vi "query_components.vi"(8 "error in (no error)":errorcluster, 9 "version":i32, 10 "part":string, 11 "DB Session ID":i32) -> (0 "error out":errorcluster, 1 "Components":T1[](array[typedef]), 3 "DB Session ID out":i32)   [LabVIEW 2023, in "Database.lvlib"]
uses:
  Database.lvlib
  DB Component.ctl
  bin/Database.dll
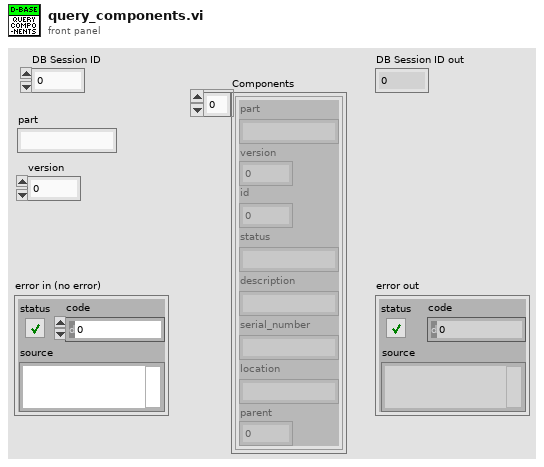
[diagram p1: front panel]
types:
  T1 = typedef "Database.lvlib/DB Component.ctl" = cluster{"part":string, "version":i32, "id":i32, "status":string, "description":string, "serial_number":string, "location":string, "parent":i32}
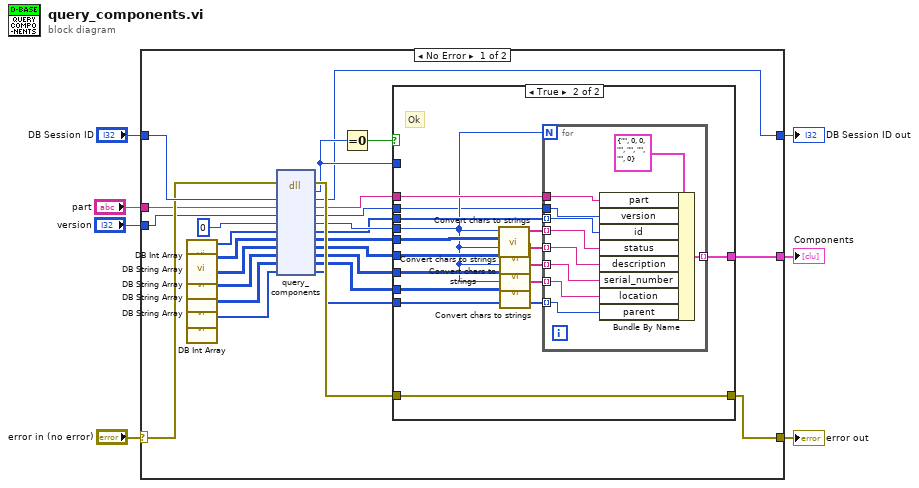
[diagram p0: block diagram]
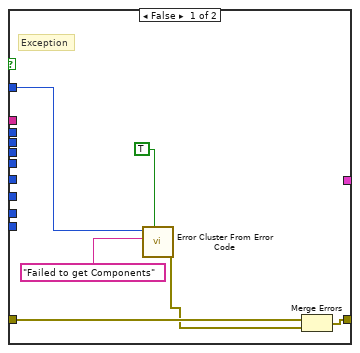
[diagram p2: hidden frame]
diagram:
  n1 = case shown="No Error" "error in (no error)" {
    selector: "error in (no error)" -> [w31 w66]
    tunnel: [w30 w66] -> w5
    tunnel: "DB Session ID" -> [w32 w65]
    tunnel: [w27 _] -> w2
    tunnel: [w25 w65] -> w4
    tunnel: "part" -> [w20 _]
    tunnel: "version" -> [w10 _]
    frame No Error {
      n2 = call "DB Int Array.vi"() -> ("DB Int Array"=w19:i32[])  [unwired: 11 in]
      n3 = call "DB String Array.vi"() -> ("DB string array"=w18:i8[][])  [unwired: 11 in]
      n4 = call "DB String Array.vi"() -> ("DB string array"=w17:i8[][])  [unwired: 11 in]
      n5 = call "DB String Array.vi"() -> ("DB string array"=w16:i8[][])  [unwired: 11 in]
      n6 = call "DB String Array.vi"() -> ("DB string array"=w15:i8[][])  [unwired: 11 in]
      n7 = call "DB Int Array.vi"() -> ("DB Int Array"=w9:i32[])  [unwired: 11 in]
      n8 = dll-call lib="C:/Users/cfangmeier3/Desktop/nebraska-silicon-lab/pixel-gantry-control/Gantry/Shared Components/bin/Database.dll" fn="query_components"(error in=w31, "session_id"=w32, "part"=w20, "version"=w10, "n_component"=0, "id"=w19, "status"=w18, "description"=w17, "serial_number"=w16, "location"=w15, "parent"=w9) -> (error out=w33:errorcluster, "return type"=w26:i32, "session_id"=w25:i32, "part"=w28:string, "version"=w12:i32, "n_component"=w24:i32, "id"=w14:i32[], "status"=w23:i8[][], "description"=w22:i8[][], "serial_number"=w21:i8[][], "location"=w13:i8[][], "parent"=w8:i32[])  [unwired: 2 in, 1 out]
      n9 = Equal To 0?(x=w26) -> (x = 0?=w29:bool)
      n10 = case shown="True" w29 {
        tunnel: w33 -> [w39 w54]
        tunnel: [w38 w54] -> w30
        tunnel: w28 -> [_ w46]
        tunnel: [_ w53] -> w27
        tunnel: w26 -> [w34 _]
        tunnel: w24 -> [_ w42]
        tunnel: w23 -> [_ w52]
        tunnel: w22 -> [_ w50]
        tunnel: w21 -> [_ w48]
        tunnel: w14 -> [_ w45]
        tunnel: w13 -> [_ w43]
        tunnel: w12 -> [_ w41]
        tunnel: w8 -> [_ w40]
        frame False {
          # "Exception"
          n11 = call <vilib>:"Error Cluster From Error Code.vi"("show call chain? (False)"=TRUE, "error message (\"\")"="Failed to get Components" ("error message (\"\")"), "error code (0)"=w34) -> ("error out"=w37:errorcluster)  [unwired: 6 in]
          n12 = Merge Errors(w39, w37) -> (w38:errorcluster)
        }
        frame True {
          # "Ok"
          n13 = call "Convert chars to strings.vi"("Char Array"=w52, "Array Length"=w42) -> ("Strings"=w51:string[])  [unwired: 9 in]
          n14 = call "Convert chars to strings.vi"("Char Array"=w50, "Array Length"=w42) -> ("Strings"=w49:string[])  [unwired: 9 in]
          n15 = call "Convert chars to strings.vi"("Char Array"=w48, "Array Length"=w42) -> ("Strings"=w47:string[])  [unwired: 9 in]
          n16 = call "Convert chars to strings.vi"("Char Array"=w43, "Array Length"=w42) -> ("Strings"=w44:string[])  [unwired: 9 in]
          n17 = for {
            N: w42 -> [_]
            tunnel: [w64] -> w53 mode=indexing
            tunnel: w51 -> [w60] mode=indexing
            tunnel: w49 -> [w59] mode=indexing
            tunnel: w47 -> [w58] mode=indexing
            tunnel: w46 -> [w62]
            tunnel: w45 -> [w61] mode=indexing
            tunnel: w44 -> [w57] mode=indexing
            tunnel: w41 -> [w56]
            tunnel: w40 -> [w55] mode=indexing
            n18 = Bundle By Name(cluster=T1 {"part"="", "version"=0, "id"=0, "status"="", "description"="", "serial_number"="", "location"="", "parent"=0} ("Cluster"), "part"=w62, "version"=w56, "id"=w61, "status"=w60, "description"=w59, "serial_number"=w58, "location"=w57, "parent"=w55) -> (w64:T1)
          }
        }
      }
    }
    frame Error {
    }
  }
  "error out" <- w5
  "DB Session ID out" <- w4
  "Components" <- w2
